vi "Screen for change password.vi"() -> ()   [LabVIEW 2022 SP3]
panel:
  out "Login 2":bool
  out "Login":bool
  in  "User Name":u16(ring)
  out "Login 4":bool
  out "Old Password":string
  out "Login 3":bool
  out "New Password":string
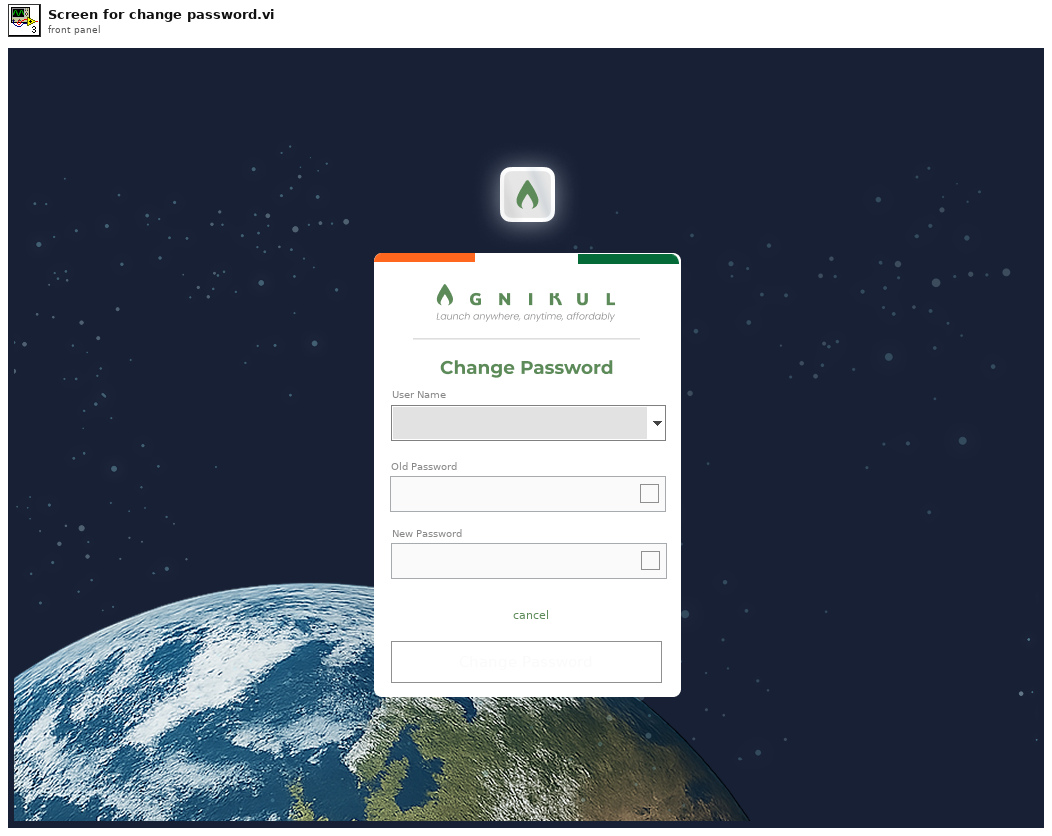
[diagram p1: front panel]
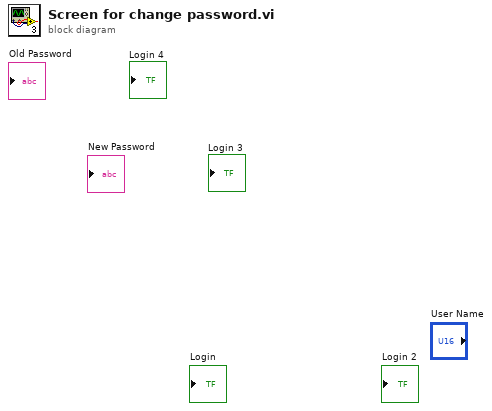
[diagram p0: block diagram]
diagram:
